vi "Set Blocksize.vi"(8 "error in":errorcluster, 10 "Blocksize":u8=16, 11 "Block Upload Transfer in":refnum<class "Block Upload Sub-Block Transfer.lvclass">) -> (0 "error out":errorcluster, 3 "Block Upload Transfer out":refnum<class "Block Upload Sub-Block Transfer.lvclass">)   [LabVIEW 2020, in "CANopen.lvlib" / "SDO Manager.lvlib" / "Block Upload Sub-Block Transfer.lvclass"]
uses:
  Block Upload Sub-Block Transfer.lvclass
  Block Upload Sub-Block Transfer.lvclass/Block Upload Sub-Block Transfer.ctl
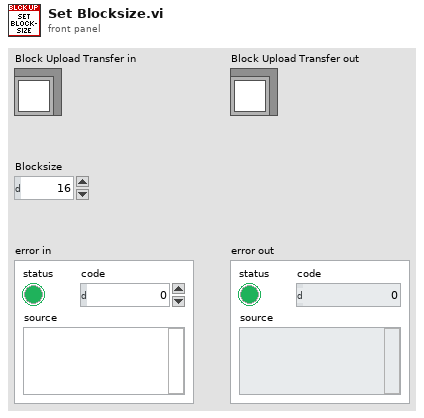
[diagram p1: front panel]
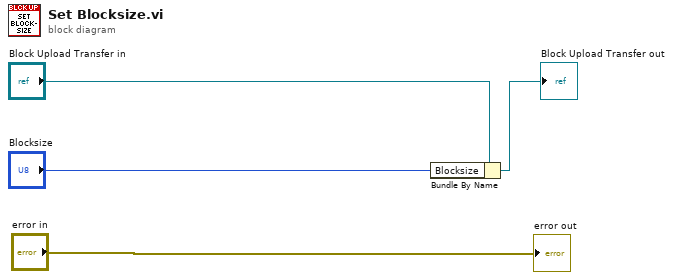
[diagram p0: block diagram]
diagram:
  n1 = Bundle By Name(cluster="Block Upload Transfer in", "Blocksize"="Blocksize") -> (→"Block Upload Transfer out":refnum<class "Block Upload Sub-Block Transfer.lvclass">)
  "error out" <- "error in"
